vi "Create_New_Build.vi"(6 "buildSpecName":string, 7 "Programmatic? (false)":bool, 8 "error in (no error)":errorcluster, 9 "buildObject":T1, 10 "Destination Path":path, 11 "AB_Deploy_EXE in":refnum<class "AB_Deploy_EXE.lvclass">) -> (0 "error out":errorcluster, 3 "AB_Deploy_EXE out":refnum<class "AB_Deploy_EXE.lvclass">)   [LabVIEW 2020, in "AB_Deploy_EXE.lvclass"]
uses:
  <vilib>/AppBuilder/AB_Classes/DeployableEXE/AB_Deploy_EXE.lvclass
  e:/builds/penguin/labview/branches/2020/dev/dist/vi.lib/AppBuilder/AB_Classes/Build/AB_Build.lvclass
  <resource>/Framework/Providers/API/ItemRef.ctl
  <vilib>/AppBuilder/AB_Classes/DeployableEXE/AB_Deploy_EXE.lvclass/AB_Deploy_EXE.ctl
  <resource>/Framework/Providers/Common/provcom_StringGlobals.vi
  <vilib>/AppBuilder/AB_Classes/EXE/AB_EXE.lvclass
  <vilib>/AppBuilder/AB_Classes/Build/AB_Build.lvclass
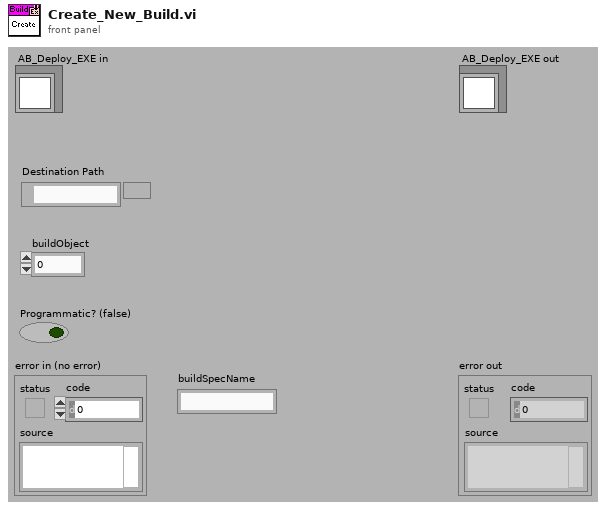
[diagram p1: front panel]
types:
  T1 = typedef "ItemRef.ctl" = u64
  T2 = typedef "AB_Build.ctl" = cluster{"buildSpecName":string, "buildSpecDescription":string, "destinations":refnum<class "AB_Destination.lvclass">[], "exclusionOption":T3, "defaultLanguage":string, "supportedLanguages":string[], "excludedDirectories":path[], "buildContext":refnum<vi>, "buildObject":T1, "preview":bool, "programatic":bool, "progressBarEvents":T4, "userLog_Path":path, "preActionID":string, "preAction_Path":path, "postActionID":string, "postAction_Path":path, "eng_checkForBrokenVIs?":bool, "eng_verboseLinkerErrors?":bool, "localDest_Path":path, "targetDest_Path":path, "removeVIObject":u16, "cache":refnum<class "PreviewCache.lvclass">, "use cache":bool, "previewCache_ID":string, "buildCache_ID":string, "eng_TempLocalDest_Path":path, "eng_collectDependencies?":bool, "versionInfo":cluster{"buildVersion":cluster{"major":u16, "minor":u16, "patch":u16, "build":u16}, "autoIncrement":bool}, "eng_enableVIChecksums":bool}
  T3 = typedef "AB_Exclusion_Option.ctl" = cluster{"typedefs":bool, "polymorphicVIs":bool, "unusedLibraryItems":bool, "modifyLibraryFile":bool, "edit-timeDependencies":bool, "inlineVIs":bool, "dependent PPLs":bool, "dependent DLLs":bool}
  T4 = typedef "provcom_ProgressBar_Events.ctl" = cluster{"newJob":refnum<user-event>, "newItem":refnum<user-event>, "errorMsg":T5, "cancel":refnum<user-event>}
  T5 = typedef "mxLvBuildError.ctl" = refnum<user-event>
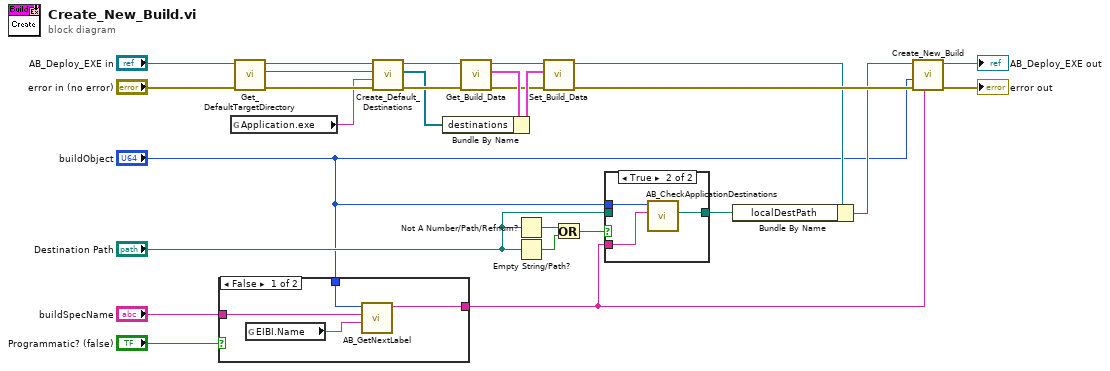
[diagram p0: block diagram]
diagram:
  n1 = case shown="False" "Programmatic? (false)" {
    tunnel: [w31 w32] -> w11
    tunnel: "buildObject" -> [w30 _]
    tunnel: "buildSpecName" -> [w29 w32]
    frame False {
      n2 = global read "provcom_StringGlobals.vi" "EIBI.Name"() -> (w28:string)
      n3 = call <vilib>:"AB_GetNextLabel.vi"("default name"=w28, "supplied name"=w29, "buildObject"=w30) -> ("New label"=w31:string)  [unwired: 3 in, 5 out]
    }
    frame True {
    }
  }
  n4 = global read "provcom_StringGlobals.vi" "Application.exe"() -> (w4:string)
  n5 = call-dynamic "Get_DefaultTargetDirectory.vi"("error in (no error)"="error in (no error)", "AB_Deploy_EXE in"="AB_Deploy_EXE in") -> ("error out"=w8:errorcluster, "default target directory"=w5:path, "AB_Deploy_EXE out"=w10:refnum<class "AB_Deploy_EXE.lvclass">)  [unwired: 7 out]
  n6 = call-dynamic "Create_Default_Destinations.vi"("error in (no error)"=w8, "Destination Name"=w4, "Destination Path"=w5, "AB_Application in"=w10) -> ("error out"=w7:errorcluster, "default dests"=w6:refnum<class "AB_Destination.lvclass">[], "AB_Application out"=w9:refnum<class "AB_Deploy_EXE.lvclass">)  [unwired: 5 out]
  n7 = call <vilib>:"Get_Build_Data.vi"("error in (no error)"=w7, "Class in"=w9) -> ("error out"=w22:errorcluster, "data"=w25:T2, "Class out"=w23:refnum<class "AB_Deploy_EXE.lvclass">)  [unwired: 7 out]
  n8 = Bundle By Name(cluster=w25, "destinations"=w6) -> (w24:T2)
  n9 = Not A Number/Path/Refnum?(number/path/refnum="Destination Path") -> (NaN/Path/Refnum?=w20:bool)
  n10 = Empty String/Path?(string/path="Destination Path") -> (empty?=w18:bool)
  n11 = call <vilib>:"Set_Build_Data.vi"("error in (no error)"=w22, "data"=w24, "Class in"=w23) -> ("error out"=w21:errorcluster, "Class out"=w17:refnum<class "AB_Deploy_EXE.lvclass">)  [unwired: 7 out]
  n12 = Or(x=w20, y=w18) -> (x .or. y?=w19:bool)
  n13 = case shown="True" w19 {
    tunnel: [w33 w34] -> w15
    tunnel: "buildObject" -> [_ w35]
    tunnel: w11 -> [_ w36]
    tunnel: "Destination Path" -> [w33 _]
    frame False {
    }
    frame True {
      n14 = call <vilib>:"AB_CheckApplicationDestinations.vi"("buildSpecName"=w36, "buildObject"=w35) -> ("Checked base path"=w34:path)  [unwired: 3 in, 6 out]
    }
  }
  n15 = Bundle By Name(cluster=w17, "localDestPath"=w15) -> (w16:refnum<class "AB_Deploy_EXE.lvclass">)
  n16 = call-parent "Create_New_Build.vi"("buildSpecName"=w11, "error in (no error)"=w21, "buildObject"="buildObject", "AB_EXE in"=w16) -> ("error out"=→"error out":errorcluster, "AB_EXE out"=→"AB_Deploy_EXE out":refnum<class "AB_Deploy_EXE.lvclass">)  [unwired: 2 in, 4 out]
